vi "Query with 1D Double Result.vi"(8 "error in (no error)":errorcluster, 10 "Query string":string, 11 "mysql in":refnum<class "mysql.lvclass">) -> (0 "error out":errorcluster, 2 "Result":dbl[](array[numeric]), 3 "mysql out":refnum<class "mysql.lvclass">)   [LabVIEW 2020, in "mysql.lvlib" / "mysql.lvclass"]
uses:
  mysql.lvclass
  0dbc43c8-e42b-42cb-9aa6-2e23bdf765e6.vi
  0dbc43c8-e42b-42cb-9aa6-2e23bdf765e6.vi/bb1e357e-4917-41ea-b5c1-45130414b1b4.vi
  0dbc43c8-e42b-42cb-9aa6-2e23bdf765e6.vi/4d31b9d5-e12b-4373-8de1-7d937d50ef3e.vi
  private/Mysql command.vi
  private/Mysql data reader 1D double.vi
  private/ping connection and reopen if needed.vi
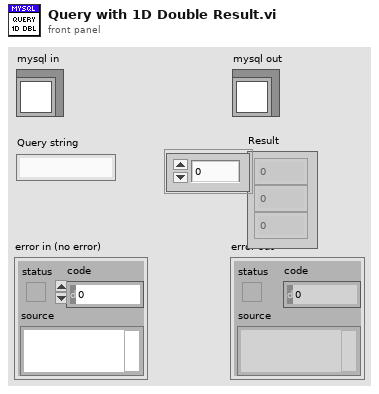
[diagram p1: front panel]
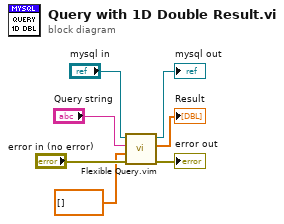
[diagram p0: block diagram]
diagram:
  n1 = call "Flexible Query.vim"("error in (no error)"="error in (no error)", "Type in"=dbl[] [] ("Result 2"), "Query string"="Query string", "mysql in"="mysql in") -> ("error out"=→"error out":errorcluster, "Result"=→"Result":dbl[], "mysql out"=→"mysql out":refnum<class "mysql.lvclass">)  [unwired: 5 in]
